vi "Autonomous Independent Chesapeake.vi"() -> ()   [LabVIEW 2011]
doc: "This VI is called when autonomous begins, and will automatically be terminated when autonomous ends. You can carry out timed or sensor driven robot movement independently without needing to return to the caller."
uses:
  <vilib>/Rock Robotics/WPI/Relay/WPI_RelayValue.ctl
  Robot Global Data.vi
  <vilib>/addons/control/pid/pid.llb/PID (DBL).vi
  <vilib>/addons/control/pid/NI_PID_pid.lvlib
panel:
  in  "Bridge Timeout (sec)":dbl=10.0
  in  "Delay for Ball 2 (sec)":ext=0.75
  out "x-y 14":dbl
  in  "Bridge Wait Time":dbl=3.0
  out "x-y 13":dbl
  out "x-y 12":dbl
  out "x-y 11":dbl
  out "x-y 10":dbl
  out "x-y 9":dbl
  out "x-y 8":dbl
  out "x-y 7":dbl
  out "x-y 6":dbl
  out "x-y 5":dbl
  out "x-y 4":dbl
  out "x-y 3":dbl
  out "x-y 2":dbl
  out "x-y":dbl
  in  "Bridge Ball Timeout (sec)":dbl=14.5
  in  "Ball 1 Timeout (sec)":dbl=6.0
  in  "Ball 2 Timeout (sec)":dbl=8.0
  out "PID Output":dbl(graph)
  in  "Deriv":dbl(knob)=0.030506642412339725 scale=0.0..0.1
  in  "Int":dbl(knob) scale=0.0..0.2
  in  "Prop":dbl(knob)=0.059181315414781936 scale=0.0..0.1
  out "RPM Control Response":cluster{"setpoint":dbl, "Angle":dbl}(graph)
  in  "Drive Brake 'Speed'":dbl=-0.25
  in  "Bridge Actuator Up Time":dbl=0.7
  in  "Bridge Shooter RPM":dbl(knob)=2375.3275564878513 scale=0.0..3000.0
  in  "Turret Yaw Control":dbl(knob)=180.7619164961486 scale=240.0..-60.0
  in  "Bridge Actuator Down Time":dbl=0.7
  in  "Drive Speed":dbl(knob)=0.9036326506562866 scale=0.0..1.0
  in  "Drive Distance (in)":dbl=46.0
  in  "Key Shooter RPM":dbl(knob)=2200.3581612281523 scale=0.0..3000.0
  # "Fire Ball 1"
  # "Shooter Stable?"
  # "Drive to Bridge"
  # "Wait for Intake"
  # "Shooter at RPM"
  # "Re-Prime for Ball 2"
  # "Fire Ball 2"
  # "Push Bridge"
  # "0.00585747"
  # "3.96963"
  # "4.19854"
  # "4.7273"
  # "6.06736"
  # "6.50122"
  # "7.63292"
  # "8.43019"
  # "14.7075"
  # "0.0028162"
  # "3.90909"
  # "4.35412"
  # "5.11691"
  # "7.55852"
  # "8.06268"
  # "9.35977"
  # "10.1718"
  # "14.7173"
  # "0.0742593"
  # "4.51218"
  # "5.00045"
  # "5.66034"
  # "7.27621"
  # "7.7194"
  # "9.01324"
  # "0"
  # "0"
  # "Cheas Match 1 was 48\""
  # "48 Inch from curve of Key to Bridge"
  # "Fairgrounds was 2415"
  # "Cheas Practice was 2325"
  # "Cheas Start was 2375"
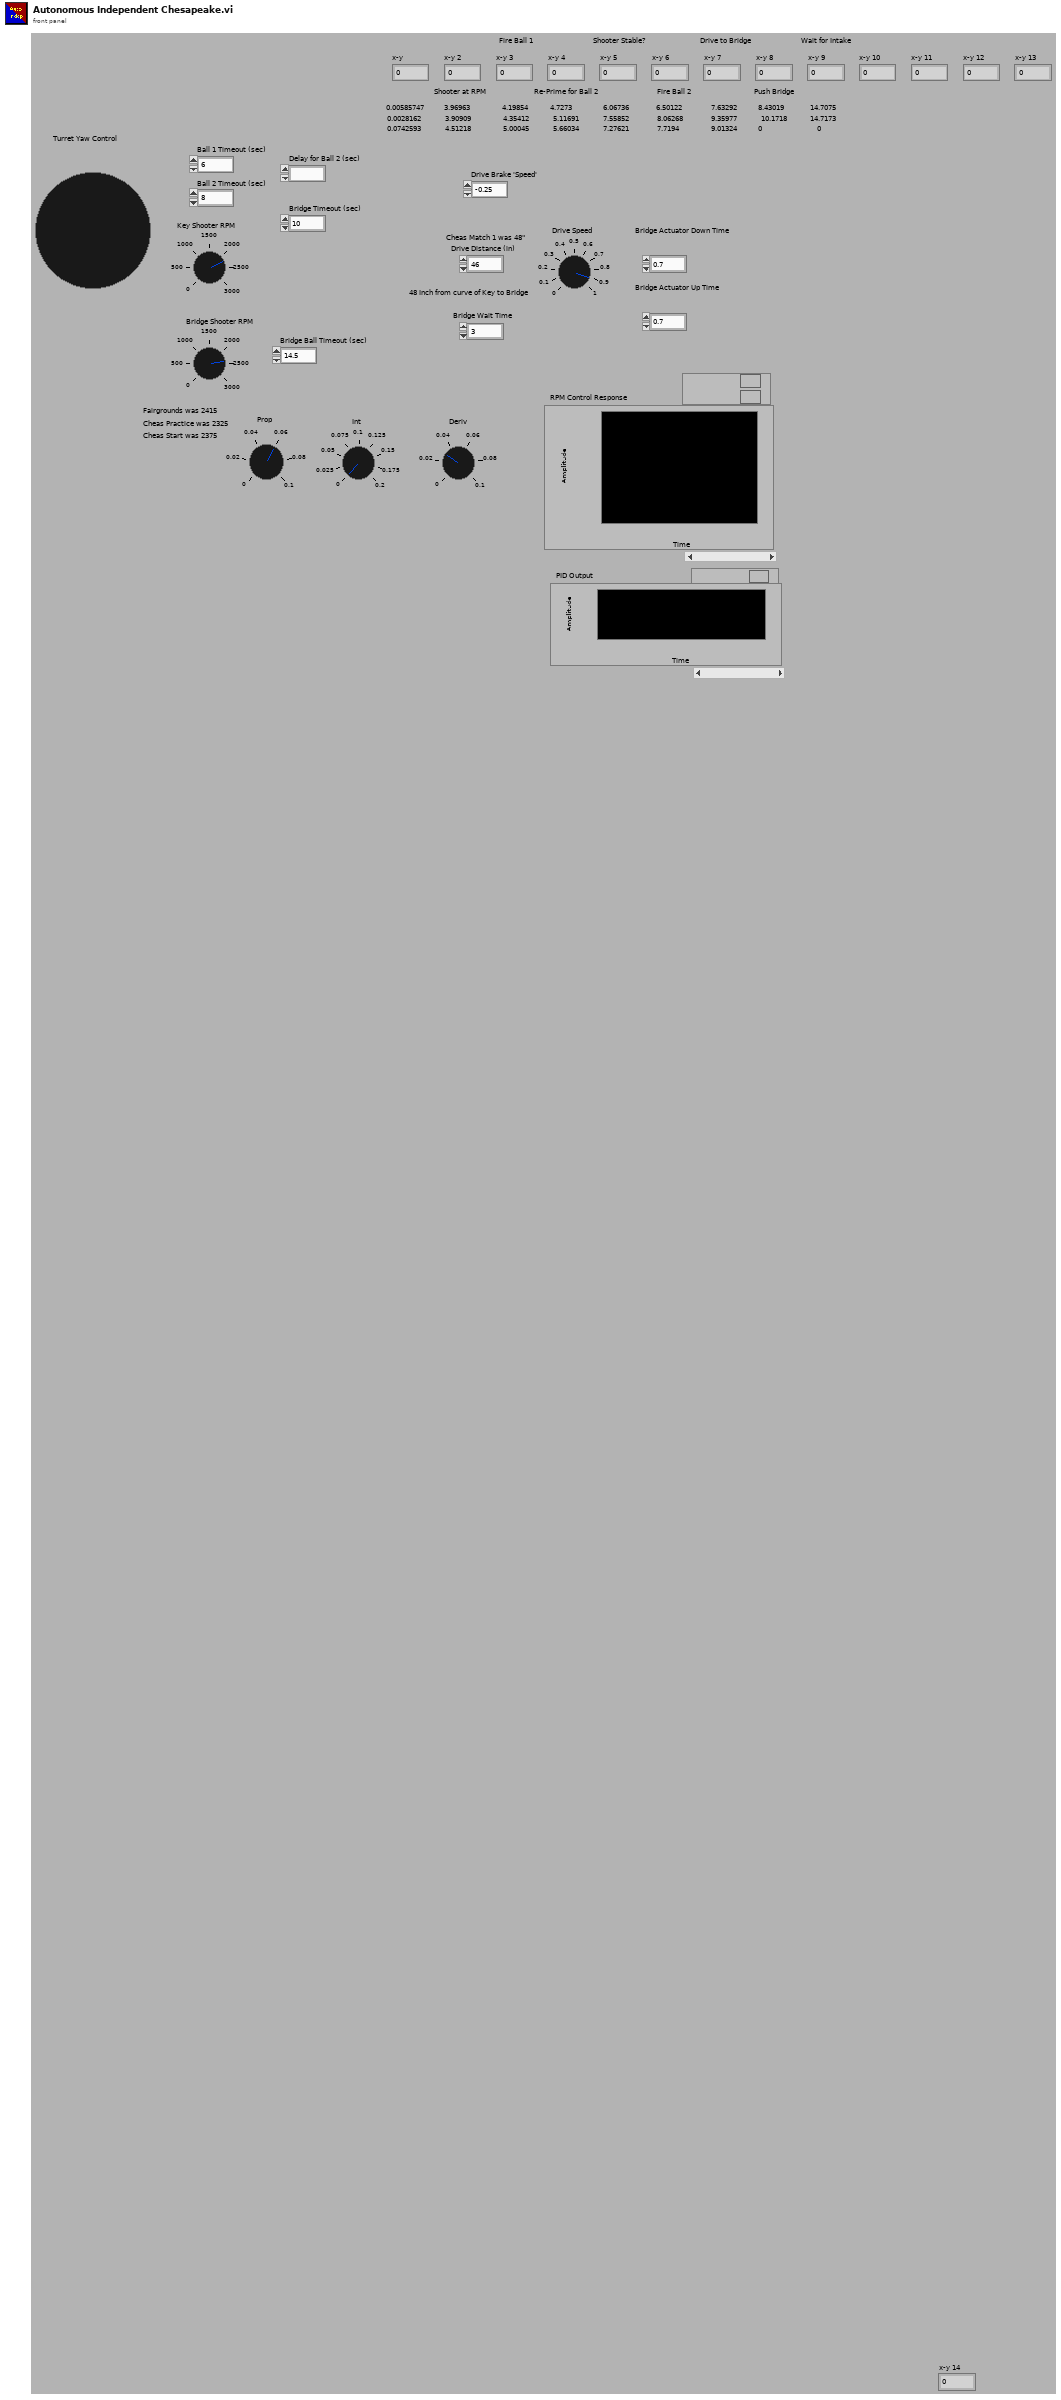
[diagram p1: front panel]
types:
  T1 = typedef "WPI_MotorControlDeviceRef.ctl" = cluster{"DeviceStatus":errorcluster, "Type":enum16{"PWM", "CAN"}, "PWM":cluster{"Digital Module":T2, "PWM Channel":T3, "DeadBand":T4}, "CAN":cluster{"Device Number":u8, "Control Mode":T5, "Semaphore":T6, "Max Vout":dbl}, "Invert":bool, "TransformRef":T7, "InvTransformRef":T7}
  T2 = typedef "FPGA_TypedefDigitalModule.ctl" = enum16{"Digital Module 1", "Digital Module 2"}
  T3 = typedef "FPGA_DIOPWMChannel.ctl" = enum8{"PWM 1", "PWM 2", "PWM 3", "PWM 4", "PWM 5", "PWM 6", "PWM 7", "PWM 8", "PWM 9", "PWM 10", "Invalid"}
  T4 = typedef "WPI_PWMDeadband.ctl" = cluster{"Name":string, "maxPositivePwm":i32, "minPositivePwm":i32, "centerPwm":i32, "maxNegativePwm":i32, "minNegativePwm":i32, "angularRange":u16}
  T5 = typedef "WPI_CANJaguar_ControlMode.ctl" = enum8{"Percent VBus", "Current", "Speed", "Position", "Voltage"}
  T6 = typedef "Semaphore RefNum" = refnum<k1>
  T7 = typedef "WPI_PWMTransform_ConPane.ctl" = refnum<vi>
  T8 = typedef "WPI_EncoderDevRef.ctl" = cluster{"DevStatus":errorcluster, "EncoderIndex":T9, "CounterIndex":T10, "DistancePerCount":dbl, "Decoding Type":T11}
  T9 = typedef "FPGA_EncoderIdx.ctl" = enum8{"Enc 0", "Enc 1", "Enc 2", "Enc 3", "Invalid"}
  T10 = typedef "FPGA_CounterCtrSystemIndex.ctl" = enum8{"Ctr 0", "Ctr 1", "Ctr 2", "Ctr 3", "Ctr 4", "Ctr 5", "Ctr 6", "Ctr 7", "Invalid"}
  T11 = typedef "WPI_EncoderType.ctl" = enum16{"1x", "2x", "4x"}
  T12 = typedef "WPI_RelayValue.ctl" = enum16{"Off", "On", "Forward", "Reverse"}
  T13 = typedef "WPI_RobotDriveDevRef.ctl" = cluster{"DevStatus":errorcluster, "Motors[]":T1[], "Square Inputs":bool, "Max Output":dbl, "Isochronous":bool}
  T14 = typedef "WPI_JoystickDevRef.ctl" = cluster{"Device":T15}
  T15 = typedef "WPI_JoystickDeviceEnum.ctl" = enum16{"USB 1", "USB 2", "USB 3", "USB 4", "Kinect 1", "Kinect 2"}
  T16 = cluster{"axis 1 (x)":dbl, "axis 2 (y)":dbl, "axis 3 (throttle)":dbl, "axis 4":dbl, "axis 5":dbl, "axis 6":dbl}
  T17 = typedef "WPI_GyroDevRef.ctl" = cluster{"DevStatus":errorcluster, "Analog Module":T18, "Analog Channel":T19, "Offset":dbl, "Gain (VoltsPerDegree/Second)":dbl}
  T18 = typedef "FPGA_TypedefAnalogModule.ctl" = enum16{"Analog Module 1", "Analog Module 2"}
  T19 = typedef "FPGA_AIChannel.ctl" = enum8{"AI 1", "AI 2", "AI 3", "AI 4", "AI 5", "AI 6", "AI 7", "AI 8", "Invalid"}
  T20 = typedef "WPI_DigitalInputDevRef.ctl" = cluster{"DevStatus":errorcluster, "DIO Channel":T21, "Digital Module":T2}
  T21 = typedef "FPGA_DIOChannel.ctl" = enum8{"DIO 1", "DIO 2", "DIO 3", "DIO 4", "DIO 5", "DIO 6", "DIO 7", "DIO 8", "DIO 9", "DIO 10", "DIO 11", "DIO 12", "DIO 13", "DIO 14", "Invalid"}
  T22 = typedef "WPI_RelayDevRef.ctl" = cluster{"DevStatus":errorcluster, "Relay Channel":T23, "Digital Module":T2, "Relay Direction":T24}
  T23 = typedef "FPGA_DIORelayChannel.ctl" = enum8{"Relay 1", "Relay 2", "Relay 3", "Relay 4", "Relay 5", "Relay 6", "Relay 7", "Relay 8", "Invalid"}
  T24 = typedef "WPI_RelayDirection.ctl" = enum16{"Both directions", "Forward only", "Reverse only"}
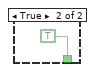
[diagram p10: hidden frame]
diagram:
  (unwired) "This code sets the toggle rate used by the Periodic Tasks VI.  For autonomous mode we slowly flash the USER1 LED on the cRIO.  Look at the Periodic Tasks VI to see how this global value is used."
  (unwired) "This function is run in parallel when the autonomous period begins. It will be terminated automatically when the period ends.\n\nNote that all Driver Station inputs are automatically latched and will not change once auto begins."
  # "Every 20ms, report that we are running autonomous\ncode. Loop will abort the same time as the VI."
  # "This gives you the joystick value\nthat is often the throttle"
  # "This tells you the driver position\nand alliance color"
  # "This gives you the eight Driver Station\ndigital switch settings"
  # "This gives you the four\nDriver Station sliders or\nanalog voltages"
  n1 = call <vilib>:"WPI_MotorControlRefNum Registry Get.vi"("refnum name"="Turret") -> ("MotorControlDevRef"=w15:T1)  [unwired: 9 in, 1 out]
  n2 = call <vilib>:"WPI_EncoderRefNum Registry Get.vi"("refnum name"="Right Wheel Encoder") -> ("EncoderDevRef"=w18:T8)  [unwired: 9 in, 1 out]
  n3 = call <vilib>:"WPI_EncoderRefNum Registry Get.vi"("refnum name"="Left Wheel Encoder") -> ("EncoderDevRef"=w19:T8)  [unwired: 9 in, 1 out]
  n4 = flat-sequence {
    tunnel: "Turret Yaw Control" -> [w35]
    tunnel: w15 -> [w36]
    tunnel: w18 -> [w37]
    tunnel: w19 -> [w38]
    tunnel: "Key Shooter RPM" -> [w39]
    tunnel: w4 -> [w32]
    tunnel: w4 -> [w44]
    tunnel: w11 -> [w62]
    tunnel: "Drive Brake 'Speed'" -> [w61]
    tunnel: w4 -> [w63]
    tunnel: w4 -> [w71]
    tunnel: w4 -> [w86]
    tunnel: w4 -> [w99]
    tunnel: w4 -> [w110]
    tunnel: w2 -> [w109]
    tunnel: w1 -> [w108]
    tunnel: w8 -> [w131]
    tunnel: w4 -> [w132]
    tunnel: w8 -> [w133]
    tunnel: "Bridge Shooter RPM" -> [w134]
    tunnel: "Drive Distance (in)" -> [w135]
    tunnel: "Drive Speed" -> [w136]
    tunnel: w11 -> [w137]
    tunnel: w11 -> [w165]
    tunnel: "Drive Brake 'Speed'" -> [w164]
    tunnel: w1 -> [w171]
    tunnel: "Bridge Actuator Down Time" -> [w172]
    tunnel: w4 -> [w170]
    tunnel: "Bridge Wait Time" -> [w190]
    tunnel: "Bridge Actuator Up Time" -> [w195]
    tunnel: w1 -> [w194]
    tunnel: w1 -> [w213]
    tunnel: w4 -> [w212]
    tunnel: w4 -> [w221]
    tunnel: w4 -> [w229]
    tunnel: w4 -> [w236]
    tunnel: "Bridge Actuator Up Time" -> [w256]
    tunnel: w1 -> [w255]
    tunnel: w4 -> [w254]
    tunnel: w1 -> [w275]
    frame #0 {
      # "Requires Collector State Machine to be\nInert in Autonomous"
      # "Initialize, start Shooter,\nand Aim Turret at Target"
      n5 = call <vilib>:"WPI_EncoderReset.vi"("EncoderDevRef"=w38) -> ()  [unwired: 9 in, 2 out]
      n6 = call <vilib>:"WPI_EncoderReset.vi"("EncoderDevRef"=w37) -> ()  [unwired: 9 in, 2 out]
      n7 = disable-structure shown="Disabled" {
        disable-tunnel: w36 -> [w42 _]
        disable-tunnel: w35 -> [w40 _]
        frame Disabled {
          n8 = call "turret.vi"("Yaw Control"=w40) -> ("Motor Output"=w41:dbl)  [unwired: 8 in, 2 out]
          n9 = call <vilib>:"WPI_MotorControlSetOutput.vi"("Output"=w41, "MotorControlDevRef"=w42) -> ()  [unwired: 8 in, 2 out]
        }
        frame Enabled {
        }
      }
      n10 = Get Date/Time In Seconds() -> (seconds since 1Jan1904=w34:timestamp)
      n11 = To Double Precision Float(number=w34) -> (double precision float=w33:dbl)
      n12 = Subtract(x=w33, y=w32) -> (x-y=→"x-y":dbl)
      n13 = global write "Robot Global Data.vi" "Shooter RPM Control"(w39) -> ()
    }
    frame #1 {
      # "May need to test for Ready & Stable,\notherwise may fire on control overshoot"
      # "Wait for Shooter to reach RPM"
      n14 = while {
        tunnel: w44 -> [w45]
        tunnel: "Ball 1 Timeout (sec)" -> [w46]
        stop <- w52 stop-if-true
        # "Timeout"
        # "Do Nothing 'til Shooter is at speed"
        n15 = global read "Robot Global Data.vi" "Shooter RPM Response"() -> (w59:dbl)
        n16 = global read "Robot Global Data.vi" "Shooter Stable?"() -> (w56:bool)
        n17 = Get Date/Time In Seconds() -> (seconds since 1Jan1904=w53:timestamp)
        n18 = To Double Precision Float(number=w53) -> (double precision float=w54:dbl)
        n19 = Subtract(x=w54, y=w45) -> (x-y=→"x-y 2":dbl)
        n20 = Greater Or Equal?(x=w59, y=1000.0) -> (x >= y?=w57:bool)
        n21 = Wait (ms)(milliseconds to wait=u32 10) -> ()  [unwired: 1 out]
        n22 = And(x=w57, y=w56) -> (x .and. y?=w48:bool)
        n23 = Get Date/Time In Seconds() -> (seconds since 1Jan1904=w50:timestamp)
        n24 = Add(x=w45, y=w46) -> (x+y=w49:dbl)
        n25 = To Double Precision Float(number=w50) -> (double precision float=w51:dbl)
        n26 = Greater Or Equal?(x=w51, y=w49) -> (x >= y?=w47:bool)
        n27 = Or(x=w47, y=w48) -> (x .or. y?=w52:bool)
      }
    }
    frame #2 {
      n28 = call <vilib>:"WPI_RobotDriveTankDrive.vi"("Right axis value"=w61, "Left axis value"=w61, "RobotDriveDevRef"=w62) -> ()  [unwired: 1 in, 8 out]
    }
    frame #3 {
      # "Will PRIME turn off too early, \nbefore ball has left the Shooter?"
      # "Fire Ball 1"
      n29 = while {
        tunnel: w63 -> [w67]
        stop <- w64 continue-if-true
        # "Fire"
        n30 = Wait (ms)(milliseconds to wait=u32 10) -> ()  [unwired: 1 out]
        n31 = global read "Robot Global Data.vi" "PRIME"() -> (w64:bool)
        n32 = Get Date/Time In Seconds() -> (seconds since 1Jan1904=w69:timestamp)
        n33 = global write "Robot Global Data.vi" "Op Button 5"(TRUE ("Op Button 5")) -> ()
        n34 = To Double Precision Float(number=w69) -> (double precision float=w68:dbl)
        n35 = Subtract(x=w68, y=w67) -> (x-y=→"x-y 3":dbl)
      }
    }
    frame #4 {
      # "Re prime for Ball 2"
      n36 = while {
        tunnel: w71 -> [w74]
        stop <- w78 stop-if-true
        # "Zach said this needs to be on"
        # "Fire Conv On"
        # "Mid Conv Forward"
        n37 = global write "Robot Global Data.vi" "Op Button 5"(TRUE ("Op Button 5")) -> ()
        n38 = Get Date/Time In Seconds() -> (seconds since 1Jan1904=w77:timestamp)
        n39 = To Double Precision Float(number=w77) -> (double precision float=w76:dbl)
        n40 = global read "Robot Global Data.vi" "PRIME"() -> (w78:bool)
        n41 = Subtract(x=w76, y=w74) -> (x-y=→"x-y 4":dbl)
        n42 = global write "Robot Global Data.vi" "Op Button 1"(TRUE ("Op Button 5")) -> ()
        n43 = Wait (ms)(milliseconds to wait=u32 10) -> ()  [unwired: 1 out]
      }
    }
    frame #5 {
      n44 = disable-structure shown="Disabled" {
        frame Disabled {
          n45 = Tick Count (ms)() -> ()  [unwired: 1 out]
        }
        frame Enabled {
        }
      }
      n46 = Multiply(x="Delay for Ball 2 (sec)", y=1000.0) -> (x*y=w82:ext)
      n47 = Wait (ms)(milliseconds to wait=w82) -> ()  [unwired: 1 out]
    }
    frame #6 {
      # "Mid Conv Off"
      # "Fire Conv Off"
      # "May need to test for Ready & Stable,\notherwise may fire on control overshoot"
      # "Stop Conveyors and Spin Up Shooter"
      # "Spin Up"
      # "Stop"
      n48 = while {
        tunnel: w86 -> [w88]
        tunnel: "Ball 2 Timeout (sec)" -> [w87]
        stop <- w90 stop-if-true
        # "Timeout"
        # "Do Nothing 'til Shooter is at speed"
        n49 = Get Date/Time In Seconds() -> (seconds since 1Jan1904=w95:timestamp)
        n50 = Wait (ms)(milliseconds to wait=u32 10) -> ()  [unwired: 1 out]
        n51 = To Double Precision Float(number=w95) -> (double precision float=w96:dbl)
        n52 = Subtract(x=w96, y=w88) -> (x-y=→"x-y 5":dbl)
        n53 = global read "Robot Global Data.vi" "Shooter Stable?"() -> (w89:bool)
        n54 = Get Date/Time In Seconds() -> (seconds since 1Jan1904=w93:timestamp)
        n55 = Add(x=w88, y=w87) -> (x+y=w92:dbl)
        n56 = To Double Precision Float(number=w93) -> (double precision float=w94:dbl)
        n57 = Greater Or Equal?(x=w94, y=w92) -> (x >= y?=w91:bool)
        n58 = Or(x=w91, y=w89) -> (x .or. y?=w90:bool)
      }
      n59 = global write "Robot Global Data.vi" "Op Button 5"(FALSE ("Op Button 5")) -> ()
      n60 = global write "Robot Global Data.vi" "Op Button 1"(FALSE ("Op Button 5")) -> ()
    }
    frame #7 {
      # "Will PRIME turn off too early, \nbefore ball has left the Shooter?"
      # "Fire Ball 2"
      n61 = while {
        tunnel: w99 -> [w103]
        stop <- w100 continue-if-true
        # "Fire"
        n62 = global write "Robot Global Data.vi" "Op Button 5"(TRUE ("Op Button 5")) -> ()
        n63 = Get Date/Time In Seconds() -> (seconds since 1Jan1904=w105:timestamp)
        n64 = global read "Robot Global Data.vi" "PRIME"() -> (w100:bool)
        n65 = To Double Precision Float(number=w105) -> (double precision float=w104:dbl)
        n66 = Subtract(x=w104, y=w103) -> (x-y=→"x-y 6":dbl)
        n67 = Wait (ms)(milliseconds to wait=u32 10) -> ()  [unwired: 1 out]
      }
    }
    frame #8 {
      n68 = global write "Robot Global Data.vi" "Dr Button 5"(TRUE ("Dr Button 5")) -> ()
      n69 = disable-structure shown="Disabled" {
        disable-tunnel: w110 -> [w114 _]
        disable-tunnel: w109 -> [w113 _]
        disable-tunnel: w108 -> [w112 _]
        frame Disabled {
          # "Push Bridge Down"
          n70 = while {
            tunnel: w114 -> [w120]
            tunnel: w113 -> [w125]
            tunnel: "Bridge Timeout (sec)" -> [w119]
            stop <- w116 stop-if-true
            # "Timeout"
            n71 = Get Date/Time In Seconds() -> (seconds since 1Jan1904=w126:timestamp)
            n72 = call <vilib>:"WPI_DigitalInputGetValue.vi"("DigitalInputDevRef"=w125) -> ("Value"=w124:bool)  [unwired: 8 in, 2 out]
            n73 = Get Date/Time In Seconds() -> (seconds since 1Jan1904=w122:timestamp)
            n74 = To Double Precision Float(number=w126) -> (double precision float=w127:dbl)
            n75 = Add(x=w120, y=w119) -> (x+y=w121:dbl)
            n76 = Not(x=w124) -> (.not. x?=w117:bool)
            n77 = To Double Precision Float(number=w122) -> (double precision float=w123:dbl)
            n78 = Subtract(x=w127, y=w120) -> (x-y=→"x-y 14":dbl)
            n79 = Greater Or Equal?(x=w123, y=w121) -> (x >= y?=w118:bool)
            n80 = Or(x=w117, y=w118) -> (x .or. y?=w116:bool)
            n81 = Wait (ms)(milliseconds to wait=u32 10) -> ()  [unwired: 1 out]
          }
          n82 = call <vilib>:"WPI_RelaySet.vi"("RelayValue"=WPI_RelayValue."Reverse", "RelayDevRef"=w112) -> ()  [unwired: 8 in, 2 out]
        }
        frame Enabled {
        }
      }
    }
    frame #9 {
      # "Fire Conv Off"
      n83 = global write "Robot Global Data.vi" "Op Button 5"(FALSE ("Op Button 5")) -> ()
      n84 = call <vilib>:"WPI_GyroReset.vi"("GyroDevRef"=w131) -> ()  [unwired: 9 in, 2 out]
    }
    frame #10 {
      # "Primitive Drive Straight Capability"
      # "Drive Straight to Coop Bridge"
      n85 = global write "Robot Global Data.vi" "Shooter RPM Control"(w134) -> ()
      n86 = while {
        tunnel: w137 -> [w161]
        tunnel: w136 -> [w146]
        tunnel: w135 -> [w158]
        tunnel: w133 -> [w149]
        tunnel: w132 -> [w138]
        stop <- w160 stop-if-true
        n87 = call <vilib>:"WPI_GyroGetAngle.vi"("GyroDevRef"=w149) -> ("Angle"=w144:dbl)  [unwired: 7 in, 3 out]
        n88 = Bundle("setpoint"=0.0, "Angle"=w144) -> (→"RPM Control Response":cluster{"setpoint":dbl, "Angle":dbl})  [unwired: 1 out]
        n89 = Get Date/Time In Seconds() -> (seconds since 1Jan1904=w141:timestamp)
        n90 = Bundle("Prop"="Prop", "Int"="Int", "Deriv"="Deriv") -> (w150:cluster{"Prop":dbl, "Int":dbl, "Deriv":dbl})  [unwired: 1 out]
        n91 = To Double Precision Float(number=w141) -> (double precision float=w140:dbl)
        n92 = global read "Robot Global Data.vi" "Avg Wheel Encoder"() -> (w159:dbl)
        n93 = Subtract(x=w140, y=w138) -> (x-y=→"x-y 7":dbl)
        n94 = Bundle("x"=0.7, -0.7) -> (w153:cluster{"x":dbl, dbl})  [unwired: 1 out]
        n95 = call-poly <vilib>:"PID.vi"("output range"=w153, "PID gains"=w150, "process variable"=w144, "setpoint"=0.0) -> ("output"=w142:dbl)  [unwired: 2 in, 5 out]
        "PID Output" <- w142
        n96 = Subtract(x=w146, y=w142) -> (x-y=w147:dbl)
        n97 = Greater Or Equal?(x=w159, y=w158) -> (x >= y?=w160:bool)
        n98 = call <vilib>:"WPI_RobotDriveTankDrive.vi"("Right axis value"=w147, "Left axis value"=w146, "RobotDriveDevRef"=w161) -> ()  [unwired: 1 in, 8 out]
        n99 = Wait (ms)(milliseconds to wait=u32 10) -> ()  [unwired: 1 out]
      }
    }
    frame #11 {
      # "Stop Drive, Brake,\nand Start up all Conveyors"
      # "Requires State Machine for more than one Ball"
      n100 = disable-structure shown="Disabled" {
        frame Disabled {
          # "Mid Conv Forward"
          # "Lo Conv Forward"
          # "Intake On"
          # "Fire Conv On"
          n101 = global write "Robot Global Data.vi" "Op Button 5"(TRUE ("Op Button 5")) -> ()
          n102 = global write "Robot Global Data.vi" "Op Button 8"(TRUE ("Op Button 5")) -> ()
          n103 = global write "Robot Global Data.vi" "Op Button 2"(TRUE ("Op Button 5")) -> ()
          n104 = global write "Robot Global Data.vi" "Op Button 1"(TRUE ("Op Button 5")) -> ()
        }
        frame Enabled {
        }
      }
      n105 = global write "Robot Global Data.vi" "Collector State Machine"(TRUE ("Collector State Machine")) -> ()
      n106 = global write "Robot Global Data.vi" "Dr Button 5"(FALSE ("Dr Button 5")) -> ()
      n107 = call <vilib>:"WPI_RobotDriveTankDrive.vi"("Right axis value"=w164, "Left axis value"=w164, "RobotDriveDevRef"=w165) -> ()  [unwired: 1 in, 8 out]
    }
    frame #12 {
      # "Actuation Time may require adjusting"
      n108 = disable-structure shown="Disabled" {
        disable-tunnel: w172 -> [w178 _]
        disable-tunnel: w171 -> [w174 _]
        disable-tunnel: w170 -> [w173 _]
        frame Disabled {
          # "Push Bridge Down"
          n109 = Get Date/Time In Seconds() -> (seconds since 1Jan1904=w176:timestamp)
          n110 = To Double Precision Float(number=w176) -> (double precision float=w177:dbl)
          n111 = while {
            tunnel: w177 -> [w187]
            tunnel: w178 -> [w186]
            tunnel: w173 -> [w179]
            stop <- w189 stop-if-true
            n112 = Get Date/Time In Seconds() -> (seconds since 1Jan1904=w180:timestamp)
            n113 = To Double Precision Float(number=w180) -> (double precision float=w181:dbl)
            n114 = Subtract(x=w181, y=w179) -> (x-y=→"x-y 8":dbl)
            n115 = Add(x=w186, y=w187) -> (x+y=w188:dbl)
            n116 = Get Date/Time In Seconds() -> (seconds since 1Jan1904=w185:timestamp)
            n117 = To Double Precision Float(number=w185) -> (double precision float=w184:dbl)
            n118 = Greater Or Equal?(x=w184, y=w188) -> (x >= y?=w189:bool)
            n119 = Wait (ms)(milliseconds to wait=u32 10) -> ()  [unwired: 1 out]
          }
          n120 = call <vilib>:"WPI_RelaySet.vi"("RelayValue"=WPI_RelayValue."Reverse", "RelayDevRef"=w174) -> ()  [unwired: 8 in, 2 out]
        }
        frame Enabled {
        }
      }
    }
    frame #13 {
      # "Wait for Bridge Balls to Roll Down Bridge\nand Magically Jump Iinto our Collector"
      n121 = disable-structure shown="Disabled" {
        disable-tunnel: w190 -> [w191 _]
        frame Disabled {
          n122 = Multiply(x=w191, y=1000.0) -> (x*y=w193:dbl)
          n123 = Wait (ms)(milliseconds to wait=w193) -> ()  [unwired: 1 out]
        }
        frame Enabled {
        }
      }
    }
    frame #14 {
      # "REMOVE IF WANT TO GO BACK TO MANUAL BRIDGE BALL FIRING"
      n124 = disable-structure shown="Disabled" {
        disable-tunnel: w195 -> [w197 _]
        disable-tunnel: w194 -> [w196 _]
        frame Disabled {
          # "Bring Bridge Actuator Up"
          n125 = Get Date/Time In Seconds() -> (seconds since 1Jan1904=w199:timestamp)
          n126 = To Double Precision Float(number=w199) -> (double precision float=w198:dbl)
          n127 = while {
            tunnel: w196 -> [w200]
            tunnel: w198 -> [w205]
            tunnel: w197 -> [w204]
            stop <- w207 stop-if-true
            n128 = Add(x=w204, y=w205) -> (x+y=w206:dbl)
            n129 = Get Date/Time In Seconds() -> (seconds since 1Jan1904=w203:timestamp)
            n130 = call <vilib>:"WPI_RelaySet.vi"("RelayValue"=WPI_RelayValue."Forward", "RelayDevRef"=w200) -> ()  [unwired: 8 in, 2 out]
            n131 = To Double Precision Float(number=w203) -> (double precision float=w202:dbl)
            n132 = Greater Or Equal?(x=w202, y=w206) -> (x >= y?=w207:bool)
            n133 = Wait (ms)(milliseconds to wait=u32 10) -> ()  [unwired: 1 out]
          }
        }
        frame Enabled {
        }
      }
    }
    frame #15 {
      # "AUTONOMOUS WILL JUST STOP HERE"
      # "REMOVE IF WANT TO GO BACK TO MANUAL BRIDGE BALL FIRING"
      n134 = while {
        stop <- FALSE stop-if-true
        # "Fire"
        n135 = global read "Robot Global Data.vi" "PRIME"() -> (w209:bool)
        n136 = global write "Robot Global Data.vi" "Op Button 5"(w209) -> ()
        n137 = Wait (ms)(milliseconds to wait=u32 10) -> ()  [unwired: 1 out]
      }
    }
    frame #16 {
      # "Wait for Intake"
      n138 = while {
        tunnel: w212 -> [w215]
        stop <- w220 stop-if-true
        n139 = Get Date/Time In Seconds() -> (seconds since 1Jan1904=w218:timestamp)
        n140 = To Double Precision Float(number=w218) -> (double precision float=w217:dbl)
        n141 = Subtract(x=w217, y=w215) -> (x-y=→"x-y 9":dbl)
        n142 = global read "Robot Global Data.vi" "INTAKE"() -> (w220:bool)
        n143 = Wait (ms)(milliseconds to wait=u32 10) -> ()  [unwired: 1 out]
      }
      n144 = call <vilib>:"WPI_RelaySet.vi"("RelayValue"=WPI_RelayValue."Off", "RelayDevRef"=w213) -> ()  [unwired: 8 in, 2 out]
    }
    frame #17 {
      # "May need to Re-Aim"
      # "May need to test for Ready & Stable,\notherwise may fire on control overshoot"
      # "Wait for Shooter to reach RPM\nand have ball PRIMEd"
      n145 = while {
        tunnel: w221 -> [w222]
        stop <- w226 stop-if-true
        # "Do Nothing 'til Shooter is at speed"
        n146 = Get Date/Time In Seconds() -> (seconds since 1Jan1904=w223:timestamp)
        n147 = To Double Precision Float(number=w223) -> (double precision float=w224:dbl)
        n148 = Subtract(x=w224, y=w222) -> (x-y=→"x-y 10":dbl)
        n149 = global read "Robot Global Data.vi" "PRIME"() -> (w226:bool)
        n150 = Wait (ms)(milliseconds to wait=u32 10) -> ()  [unwired: 1 out]
      }
    }
    frame #18 {
      # "Fire Conv Off"
      n151 = while {
        tunnel: w229 -> [w230]
        stop <- w235 stop-if-true
        n152 = Get Date/Time In Seconds() -> (seconds since 1Jan1904=w233:timestamp)
        n153 = To Double Precision Float(number=w233) -> (double precision float=w232:dbl)
        n154 = Subtract(x=w232, y=w230) -> (x-y=→"x-y 11":dbl)
        n155 = global read "Robot Global Data.vi" "Shooter Stable?"() -> (w235:bool)
        n156 = Wait (ms)(milliseconds to wait=u32 10) -> ()  [unwired: 1 out]
      }
      n157 = global write "Robot Global Data.vi" "Op Button 5"(FALSE ("Op Button 5")) -> ()
    }
    frame #19 {
      # "Will PRIME turn off too early, \nbefore ball has left the Shooter?"
      # "Fire Bridge Ball 1"
      n158 = while {
        tunnel: "Bridge Ball Timeout (sec)" -> [w242]
        tunnel: w236 -> [w240]
        stop <- w243 stop-if-true
        # "Fire"
        n159 = global write "Robot Global Data.vi" "Op Button 5"(TRUE ("Op Button 5")) -> ()
        n160 = global read "Robot Global Data.vi" "PRIME"() -> (w246:bool)
        n161 = Wait (ms)(milliseconds to wait=u32 10) -> ()  [unwired: 1 out]
        n162 = Not(x=w246) -> (.not. x?=w245:bool)
        n163 = Get Date/Time In Seconds() -> (seconds since 1Jan1904=w248:timestamp)
        n164 = Add(x=w240, y=w242) -> (x+y=w247:dbl)
        n165 = To Double Precision Float(number=w248) -> (double precision float=w241:dbl)
        n166 = Greater Or Equal?(x=w241, y=w247) -> (x >= y?=w244:bool)
        n167 = Subtract(x=w241, y=w240) -> (x-y=→"x-y 12":dbl)
        n168 = Or(x=w244, y=w245) -> (x .or. y?=w243:bool)
      }
    }
    frame #20 {
      # "Mid Conv Forward"
      # "Lo Conv Forward"
      # "Fire Conv Off"
      # "Stop all Conveyors"
      n169 = global write "Robot Global Data.vi" "Op Button 2"(FALSE ("Op Button 5")) -> ()
      n170 = global write "Robot Global Data.vi" "Op Button 1"(FALSE ("Op Button 5")) -> ()
      n171 = global write "Robot Global Data.vi" "Op Button 5"(FALSE ("Op Button 5")) -> ()
      n172 = global write "Robot Global Data.vi" "Op Button 8"(FALSE ("Op Button 5")) -> ()
      n173 = disable-structure shown="Disabled" {
        disable-tunnel: w256 -> [w259 _]
        disable-tunnel: w255 -> [w258 _]
        disable-tunnel: w254 -> [w257 _]
        frame Disabled {
          # "Intake Off"
          # "Bring Bridge Actuator Up"
          n174 = Get Date/Time In Seconds() -> (seconds since 1Jan1904=w261:timestamp)
          n175 = To Double Precision Float(number=w261) -> (double precision float=w260:dbl)
          n176 = while {
            tunnel: w258 -> [w266]
            tunnel: w260 -> [w271]
            tunnel: w259 -> [w270]
            tunnel: w257 -> [w262]
            stop <- w273 stop-if-true
            n177 = Get Date/Time In Seconds() -> (seconds since 1Jan1904=w265:timestamp)
            n178 = To Double Precision Float(number=w265) -> (double precision float=w264:dbl)
            n179 = Subtract(x=w264, y=w262) -> (x-y=→"x-y 13":dbl)
            n180 = Add(x=w270, y=w271) -> (x+y=w272:dbl)
            n181 = Get Date/Time In Seconds() -> (seconds since 1Jan1904=w269:timestamp)
            n182 = call <vilib>:"WPI_RelaySet.vi"("RelayValue"=WPI_RelayValue."Forward", "RelayDevRef"=w266) -> ()  [unwired: 8 in, 2 out]
            n183 = To Double Precision Float(number=w269) -> (double precision float=w268:dbl)
            n184 = Greater Or Equal?(x=w268, y=w272) -> (x >= y?=w273:bool)
            n185 = Wait (ms)(milliseconds to wait=u32 10) -> ()  [unwired: 1 out]
          }
        }
        frame Enabled {
        }
      }
    }
    frame #21 {
      n186 = global write "Robot Global Data.vi" "Collector State Machine"(TRUE ("Collector State Machine")) -> ()
      n187 = call <vilib>:"WPI_RelaySet.vi"("RelayValue"=WPI_RelayValue."Off", "RelayDevRef"=w275) -> ()  [unwired: 8 in, 2 out]
    }
    frame #22 {
      n188 = while {
        stop <- FALSE stop-if-true
        # "Fire"
        n189 = global read "Robot Global Data.vi" "PRIME"() -> (w280:bool)
        n190 = case shown="False" w280 {
          tunnel: [FALSE TRUE ("Op Button 5")] -> w279
          frame False {
          }
          frame True {
          }
        }
        n191 = global write "Robot Global Data.vi" "Op Button 5"(w279) -> ()
        n192 = Wait (ms)(milliseconds to wait=u32 10) -> ()  [unwired: 1 out]
      }
    }
  }
  n193 = Get Date/Time In Seconds() -> (seconds since 1Jan1904=w7:timestamp)
  n194 = To Double Precision Float(number=w7) -> (double precision float=w4:dbl)
  n195 = call <vilib>:"WPI_RobotDriveRefNum Registry Get.vi"("refnum name"="RobotDrive") -> ("RobotDriveDevRef"=w11:T13)  [unwired: 9 in, 1 out]
  n196 = while {
    stop <- FALSE stop-if-true
    n197 = call <vilib>:"WPI_DriverStationReport Robot Code State.vi"("Autonomous"=TRUE) -> ()  [unwired: 10 in, 1 out]
    n198 = Wait (ms)(milliseconds to wait=u32 20) -> ()  [unwired: 1 out]
  }
  n199 = call <vilib>:"WPI_DriverStationGet Alliance Info.vi"() -> ()  [unwired: 12 out]
  n200 = call <vilib>:"WPI_DriverStationGet Digital Input.vi"() -> ("Driver Station Digital Input (1-8)"=w30:bool[])  [unwired: 11 out]
  n201 = call <vilib>:"WPI_DriverStationGet Analog Input.vi"() -> ()  [unwired: 12 out]
  n202 = call <vilib>:"WPI_JoystickRefNum Registry Get.vi"("refnum name"="Joystick 1") -> ("JoystickDevRef"=w27:T14)  [unwired: 1 in, 9 out]
  n203 = call <vilib>:"WPI_JoystickGet.vi"("JoystickDevRef"=w27) -> ("Axes"=w28:T16)  [unwired: 1 in, 5 out]
  n204 = Unbundle By Name(w28) -> ()  [unwired: 1 out]
  n205 = Index Array(array=w30) -> ()  [unwired: 8 in, 8 out]
  n206 = global write "Robot Global Data.vi" "LED toggle rate (ms)"(u32 500 ("LED ms toggle rate")) -> ()
  n207 = call <vilib>:"WPI_GyroRefNum Registry Get.vi"("refnum name"="Robot Gyro") -> ("GyroDevRef"=w8:T17)  [unwired: 9 in, 1 out]
  n208 = call <vilib>:"WPI_DigitalInputRefNum Registry Get.vi"("refnum name"="Bridge Actuator Down") -> ("DigitalInputDevRef"=w2:T20)  [unwired: 9 in, 1 out]
  n209 = call <vilib>:"WPI_RelayRefNum Registry Get.vi"("refnum name"="Bridge Actuator") -> ("RelayDevRef"=w1:T22)  [unwired: 9 in, 1 out]
